vi "OphirTestMeasure_LB.vi"() -> ()   [LabVIEW 2012]
uses:
  <vilib>/Analysis/baseanly.llb/Mean (DBL).vi
  <vilib>/Analysis/NI_AALBase.lvlib
panel:
  out "output cluster":cluster{"Timeout":bool, "LB Error":bool}
  out "Power Arr":dbl[](array[numeric])
  out "Power,uW":dbl
  out "error out":errorcluster
  out "Error":bool
  in  "error in (no error)":errorcluster
  out "Units":string
  out "Frame Output":string
  out "Frame Output 2":string
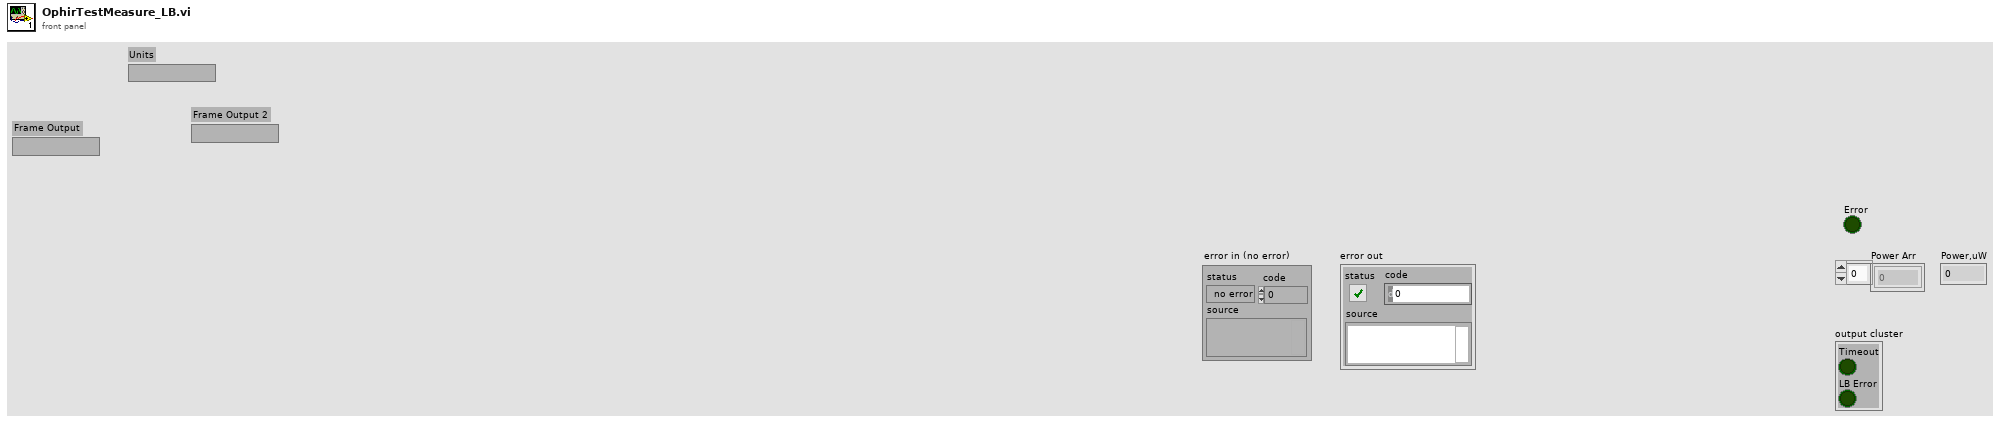
[diagram p1: front panel]
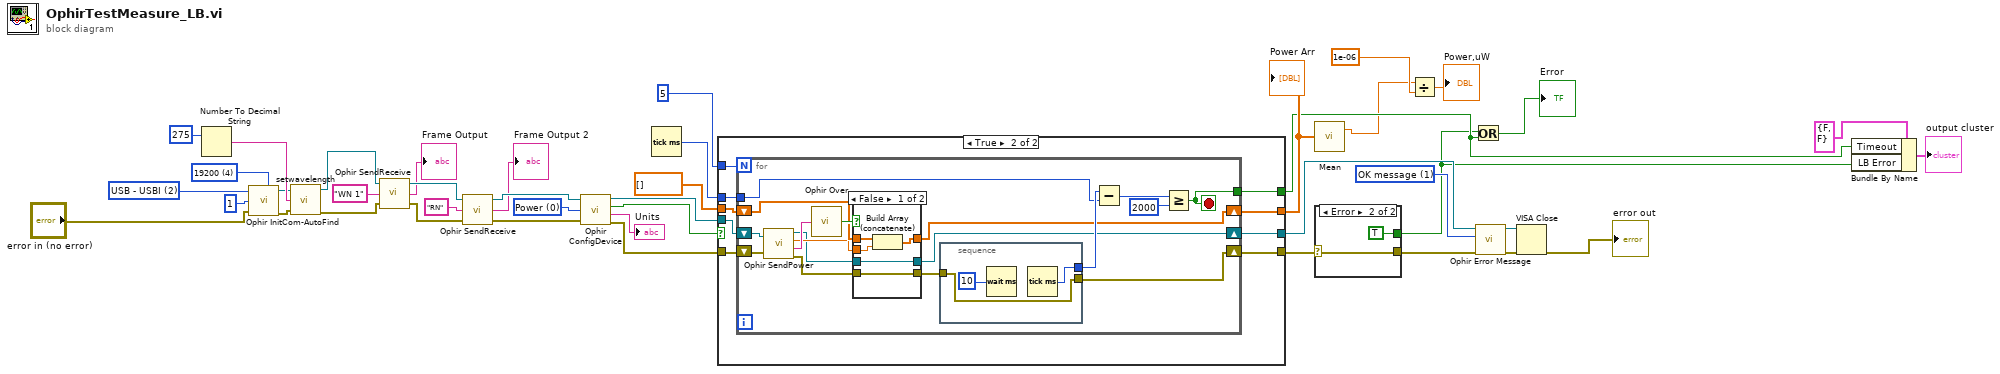
[diagram p0: block diagram]
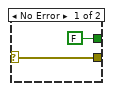
[diagram p2: hidden frame]
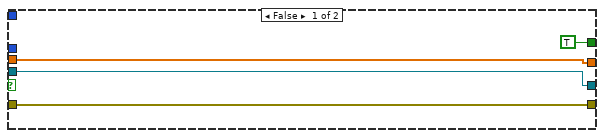
[diagram p3: hidden frame]
diagram:
  w17 = 1 items=["no dialog", "OK message", "continue or stop message"] ("Type of Dialog (OK msg:1)")
  w24 = i16 4 items=["300", "1200", "4800", "9600", "19200", "38400"] ("Baud Rate (3:9600)")
  w26 = i16 2 items=["USB - Nova2", "USB - Vega", "USB - USBI", "RS232", "GPIB"] ("communication")
  w37 = u16 0 items=["Power", "Energy", "Frequency"] ("Measure Choice (0:Power)")
  n1 = Number To Decimal String(number=275) -> (decimal integer string=w30:string)  [unwired: 1 in]
  n2 = call "Ophir InitCom-AutoFind.vi"("Baud Rate (3:9600)"=w24, "communication"=w26, "Port Number (default 2)"=i16 1, "error in (no error)"="error in (no error)") -> ("Dup Visa Session"=w22:refnum<visa-resource-name>, "error out"=w23:errorcluster)  [unwired: 2 out]
  n3 = call "setwavelength.vi"("Dup Visa Session"=w22, "Set Wavelength"=w30, "error in (no error)"=w23) -> ("dup Visa Session"=w41:refnum<visa-resource-name>, "error out"=w40:errorcluster)  [unwired: 3 in]
  n4 = call "Ophir SendReceive.vi"("error in (no error)"=w40, "Command"="WN 1", "Visa Session"=w41) -> ("error out"=w27:errorcluster, "Frame Output"=→"Frame Output":string, "dup Visa Session"=w39:refnum<visa-resource-name>)
  n5 = call "Ophir SendReceive.vi"("error in (no error)"=w27, "Command"="RN", "Visa Session"=w39) -> ("error out"=w35:errorcluster, "Frame Output"=→"Frame Output 2":string, "dup Visa Session"=w36:refnum<visa-resource-name>)
  n6 = call "Ophir ConfigDevice.vi"("Visa Session"=w36, "Measure Choice (0:Power)"=w37, "error in (no error)"=w35) -> ("dup Visa Session"=w32:refnum<visa-resource-name>, "OK ?"=w34:bool, "Units"=→"Units":string, "error out"=w33:errorcluster)
  n7 = Tick Count (ms)() -> (millisecond timer value=w28:u32)
  n8 = case shown="True" w34 {
    tunnel: w33 -> [w45 w53]
    tunnel: w32 -> [w46 w54]
    tunnel: dbl[] [] -> [w44 w55]
    tunnel: [w46 w52] -> w18
    tunnel: [w45 w51] -> w29
    tunnel: [w44 w50] -> w13
    tunnel: w28 -> [_ w49]
    tunnel: [TRUE w48] -> w11
    tunnel: 5 -> [_ w47]
    frame False {
    }
    frame True {
      n9 = for {
        N: w47 -> [_]
        shift-right: [w63] -> w50
        shift-left: w55 -> [w64]
        shift-right: [w61] -> w52
        shift-left: w54 -> [w72]
        shift-right: [w57] -> w51
        shift-left: w53 -> [w71]
        tunnel: w49 -> [w68]
        tunnel: [w56] -> w48
        stop <- w56 stop-if-true
        n10 = call "Ophir SendPower.vi"("Visa Session"=w72, "error in (no error)"=w71) -> ("dup Visa Session"=w60:refnum<visa-resource-name>, "Value Number"=w62:dbl, "Value String"=w70:string, "error out"=w58:errorcluster)
        n11 = call "Ophir Over.vi"("Value String"=w70) -> ("Overrange"=w65:bool)
        n12 = case shown="False" w65 {
          tunnel: w64 -> [w77 w80]
          tunnel: [w74 w80] -> w63
          tunnel: w62 -> [w76 _]
          tunnel: [w75 w79] -> w61
          tunnel: w60 -> [w75 w79]
          tunnel: [w73 w78] -> w59
          tunnel: w58 -> [w73 w78]
          frame False {
            n13 = Build Array (concatenate)(w77, w76) -> (w74:dbl[])
          }
          frame True {
          }
        }
        n14 = stacked-sequence {
          tunnel: [w83] -> w69
          tunnel: w59 -> [w82]
          tunnel: [w82] -> w57
          frame #0 {
            n15 = Wait (ms)(milliseconds to wait=u32 10) -> ()  [unwired: 1 out]
            n16 = Tick Count (ms)() -> (millisecond timer value=w83:u32)
          }
        }
        n17 = Subtract(x=w69, y=w68) -> (x-y=w67:u32)
        n18 = Greater Or Equal?(x=w67, y=u32 2000) -> (x >= y?=w56:bool)
      }
    }
  }
  "Power Arr" <- w13
  n19 = call-poly <vilib>:"Mean.vi"("X"=w13) -> ("mean"=w3:dbl)  [unwired: 1 out]
  n20 = case shown="Error" w29 {
    selector: w29 -> [w85 w86]
    tunnel: [w85 w86] -> w19
    tunnel: [FALSE ("x") TRUE ("x")] -> w10
    frame No Error {
    }
    frame Error {
    }
  }
  n21 = Divide(x=w3, y=1e-06) -> (x/y=→"Power,uW":dbl)
  n22 = Or(x=w10, y=w11) -> (x .or. y?=→"Error":bool)
  n23 = call "Ophir Error Message.vi"("error in (no error)"=w19, "Type of Dialog (OK msg:1)"=w17, "Visa Session"=w18) -> ("error out"=w20:errorcluster, "dup Visa Session"=w21:refnum<visa-resource-name>)  [unwired: 1 in, 2 out]
  n24 = VISA Close(VISA resource name=w21, error in (no error)=w20) -> (error out=→"error out":errorcluster)
  n25 = Bundle By Name(cluster=cluster{"Timeout":bool, "LB Error":bool} {"Timeout"=FALSE, "LB Error"=FALSE} ("Ophir Error"), "Timeout"=w11, "LB Error"=w10) -> (→"output cluster":cluster{"Timeout":bool, "LB Error":bool})
